vi "Stop.vi"(0 "eye scan in":refnum<class "niHighSpeedSerial Eye Scan v1 Host.lvclass">, 11 "error in":errorcluster) -> (4 "eye scan out":refnum<class "niHighSpeedSerial Eye Scan v1 Host.lvclass">, 15 "error out":errorcluster)   [LabVIEW 2014, in "niHighSpeedSerial Eye Scan v1 Host.lvclass"]
doc: "Stops the current measurement and transitions the session into the Aborted state. Once <b>Stop</b> is called, you cannot call <b>Measure</b> until after <b>Start</b> is called first.\n\n<B>Input Parameters</B>\n\n<B>eye scan in</B> Takes in a reference to your session from the previous VI.\n\n<B>error in</B> describes error conditions that occur before this node runs. This input provides standard 'error in' functionality.\n\n<B>Output Parameters</B>\n\n<B>eye scan out</B> passes a reference to your session to the next VI.\n\n<B>error out</B> contains error information. This output provides standard 'error out' functionality."
uses:
  <instrlib>/niHighSpeedSerial/Eye Scan/v1/Host/Eye Scan/niHighSpeedSerial Eye Scan v1 Host.lvclass
  <instrlib>/niHighSpeedSerial/Eye Scan/v1/Host/Eye Scan/niHighSpeedSerial Eye Scan v1 Host.lvclass/niHighSpeedSerial Eye Scan v1 Host.ctl
  <instrlib>/niHighSpeedSerial/Eye Scan/v1/Host/Eye Scan/Private/Measure State.ctl
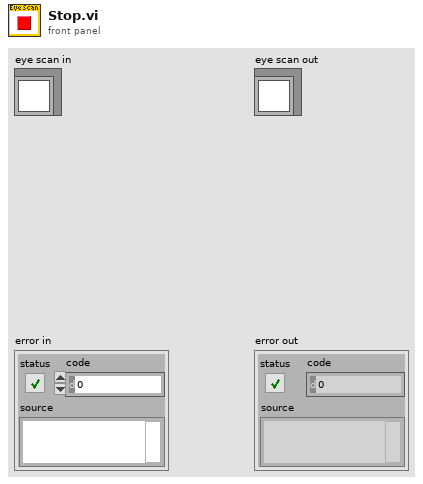
[diagram p1: front panel]
types:
  T1 = typedef "niHighSpeedSerial Eye Scan v1 Host.lvclass/Measure State.ctl" = enum16{"Uninitialized", "Initialized", "Ready", "Measuring", "Finished", "Aborted"}
  T2 = typedef "niHighSpeedSerial Eye Scan v1 Host.lvclass/Private Data.ctl" = cluster{"instruction target":refnum<class "niInstr Instruction Target v1 Host.lvclass">, "channels":T3[], "measure state":T1, "rx output divider":T4, "equalization mode":T5, "rx data width":T6, "BER floor":dbl, "number of points completed":i32, "rx output divider configured?":bool, "equalization mode configured?":bool, "rx data width configured?":bool}
  T3 = typedef "niHighSpeedSerial Eye Scan v1 Host.lvclass/Channel Data.ctl" = cluster{"instance":u8, "channel":refnum<class "niHighSpeedSerial Eye Scan Single Point v1 Host.lvclass">, "point iterator":refnum<class "niHighSpeedSerial Eye Scan Point Iterator v1 Host.lvclass">}
  T4 = typedef "niHighSpeedSerial Eye Scan Common v1 Host.lvlib/RX Output Divider.ctl" = enum16{"1", "2", "4", "8", "16"}
  T5 = typedef "niHighSpeedSerial Eye Scan Common v1 Host.lvlib/Equalization Mode.ctl" = enum16{"DFE", "LPM"}
  T6 = typedef "niHighSpeedSerial Eye Scan Common v1 Host.lvlib/Data Width.ctl" = enum16{"16 Bit", "20 Bit", "32 Bit", "40 Bit"}
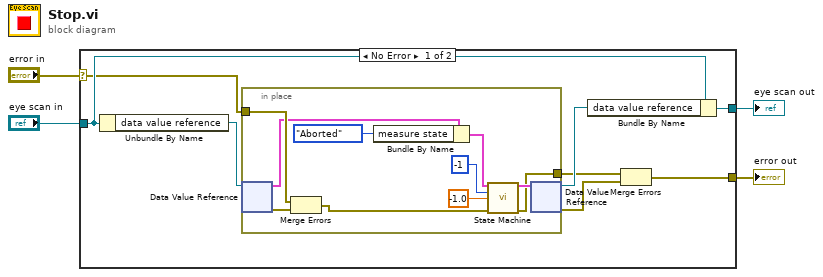
[diagram p0: block diagram]
diagram:
  n1 = case shown="No Error" "error in" {
    selector: "error in" -> [w8 w24]
    tunnel: [w5 w24] -> w3
    tunnel: [w12 w23] -> w2
    tunnel: "eye scan in" -> [w11 w23]
    frame No Error {
      n2 = Unbundle By Name(w11) -> ("data value reference"=w10:refnum<data-value>)
      n3 = in-place {
        in-place-border: w8 -> [w21]
        in-place-border: [w15] -> w6
        n4 = in-place-dvr #1(w10) -> (w19:T2, w22:errorcluster)
        n5 = Merge Errors(w21, w22) -> (w20:errorcluster)
        n6 = Bundle By Name(cluster=w19, "measure state"=Measure_State."Aborted" ("Measure State")) -> (w17:T2)
        n7 = call <instrlib>:"State Machine.vi"("private data"=w17, "requested number of new points"=-1 ("requested number of points"), "timeout (100 ms)"=-1.0, "error in"=w20) -> ("private data out"=w16:T2, "error out"=w15:errorcluster)  [unwired: 7 in, 3 out]
        n8 = in-place-dvr #1(w16) -> (w9:refnum<data-value>, w7:errorcluster)
      }
      n9 = Bundle By Name(cluster=w11, "data value reference"=w9) -> (w12:refnum<class "niHighSpeedSerial Eye Scan v1 Host.lvclass">)
      n10 = Merge Errors(w6, w7) -> (w5:errorcluster)
    }
    frame Error {
    }
  }
  "error out" <- w3
  "eye scan out" <- w2
